vi "NT Writer.vi"() -> ()   [LabVIEW 2015]
uses:
  NT Variable TypeDef.ctl
  <vilib>/Rock Robotics/Network Tables/NT Write Number.vi
  <vilib>/Rock Robotics/Network Tables/NT Write Boolean.vi
  <vilib>/Rock Robotics/Network Tables/NT Write String.vi
  <vilib>/Rock Robotics/Network Tables/NT Write Boolean Array.vi
  <vilib>/Rock Robotics/Network Tables/NT Write Numeric Array.vi
  <vilib>/Rock Robotics/Network Tables/NT Write String Array.vi
panel:
  in  "Write":bool
  in  "PID":cluster{"Kp":dbl, "Ki":dbl, "Kd":dbl}
  in  "String Array":string[](array[string])
  in  "String":string
  in  "Numeric Array":dbl[](array[numeric])
  in  "Numeric":dbl
  in  "Boolean Array":bool[](array[boolean])
  in  "stop":bool
  in  "Boolean":bool
  in  "NT Variable":u16(ring) items=["/Robot Parameters/Arm Parameters/Position Sensor Calibration/Voltage @ Max Angle (v)", "/Robot Parameters/Arm Parameters/Position Sensor Calibration/Voltage @ Min Angle (v)", "/Robot Parameters/Arm Parameters/Position Sensor Calibration/Max Angle (°)", "/Robot Parameters/Arm Parameters/Position Sensor Calibration/Min Angle (°)", "/Robot Parameters/Arm Parameters/Arm angle tolerance to lock (+|-°)", "/Robot Parameters/Drive Parameters/Default Orientation (F-Normal; T-Reversed)", "/Robot Parameters/Intake Parameters/Suck-in Speed (-1 to 1)", "/Robot Parameters/Intake Parameters/Spit-out Speed (-1 to 1)", "/Robot Parameters/Arm Parameters/Auto Arm Up Speed (in per s)", "/Robot Parameters/Arm Parameters/Position Sensor Calibration/Min Angle (°)", "/Robot Parameters/Arm Parameters/Position Sensor Calibration/Max Angle (°)", "/Robot Parameters/Arm Parameters/Driver Cross Defense Angle  (90° - 180°)", "/Robot Parameters/Drive Parameters/Reduced Speed Gain (0-1)", "/Robot Parameters/Arm Parameters/Arm Motor PID Gains", "/Robot Parameters/Shooter Parameters/Shoot Solenoid Time (ms)", "/Robot Parameters/Shooter Parameters/Open Claw Time (ms)", "/Robot Parameters/Shooter Parameters/Pressure threshold for shooting (PSI)", "/Robot Parameters/Drive Parameters/IMU PID Gains", "/Robot Parameters/Drive Parameters/Encoder PID Gains", "/Robot Parameters/Drive Parameters/GRIP PID Gains", "/Robot Parameters/Shooter Parameters/Arm angle threshold for shooting (90°-180°)", "/Robot Parameters/Drive Parameters/Slew Rate (Units per Second)", "/Robot Parameters/Drive Parameters/Joystick Configuration (0 - Split Axis Arcade; 1 - Arcade; 2 - Tank)", "/Robot Parameters/Arm Parameters/Presets/Shoot Batter (°, Lock)", "/Robot Parameters/Arm Parameters/Presets/Shoot Close (°, Lock)", "/Robot Parameters/Arm Parameters/Presets/Cross Defense (°, Lock)", "/Robot Parameters/Arm Parameters/Presets/Human Player Load (°, Lock)", "/Robot Parameters/Arm Parameters/Presets/Low Bar, Low Goal (°, Lock)"]
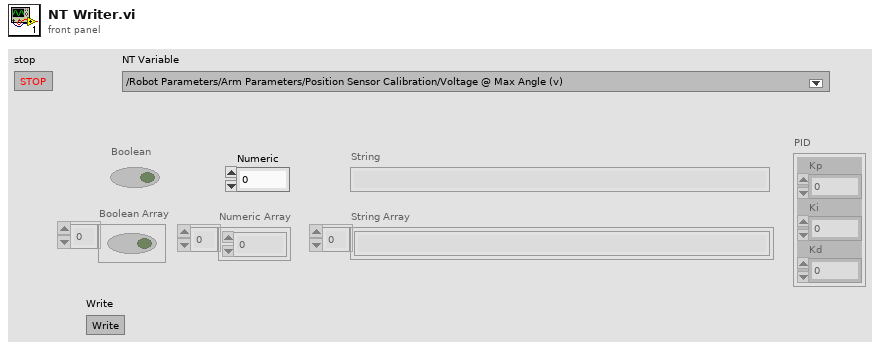
[diagram p1: front panel]
types:
  T1 = typedef "NT Variable TypeDef.ctl" = cluster{"NT Variable Name":string, "NT Type":enum16{"Boolean", "Numeric", "String", "Boolean Array", "Numeric Array", "String Array", "PID"}}
  T2 = enum8{"Enabled", "Disabled", "Disabled and Grayed Out"}
  T3 = enum16{"Boolean", "Numeric", "String", "Boolean Array", "Numeric Array", "String Array", "PID"}
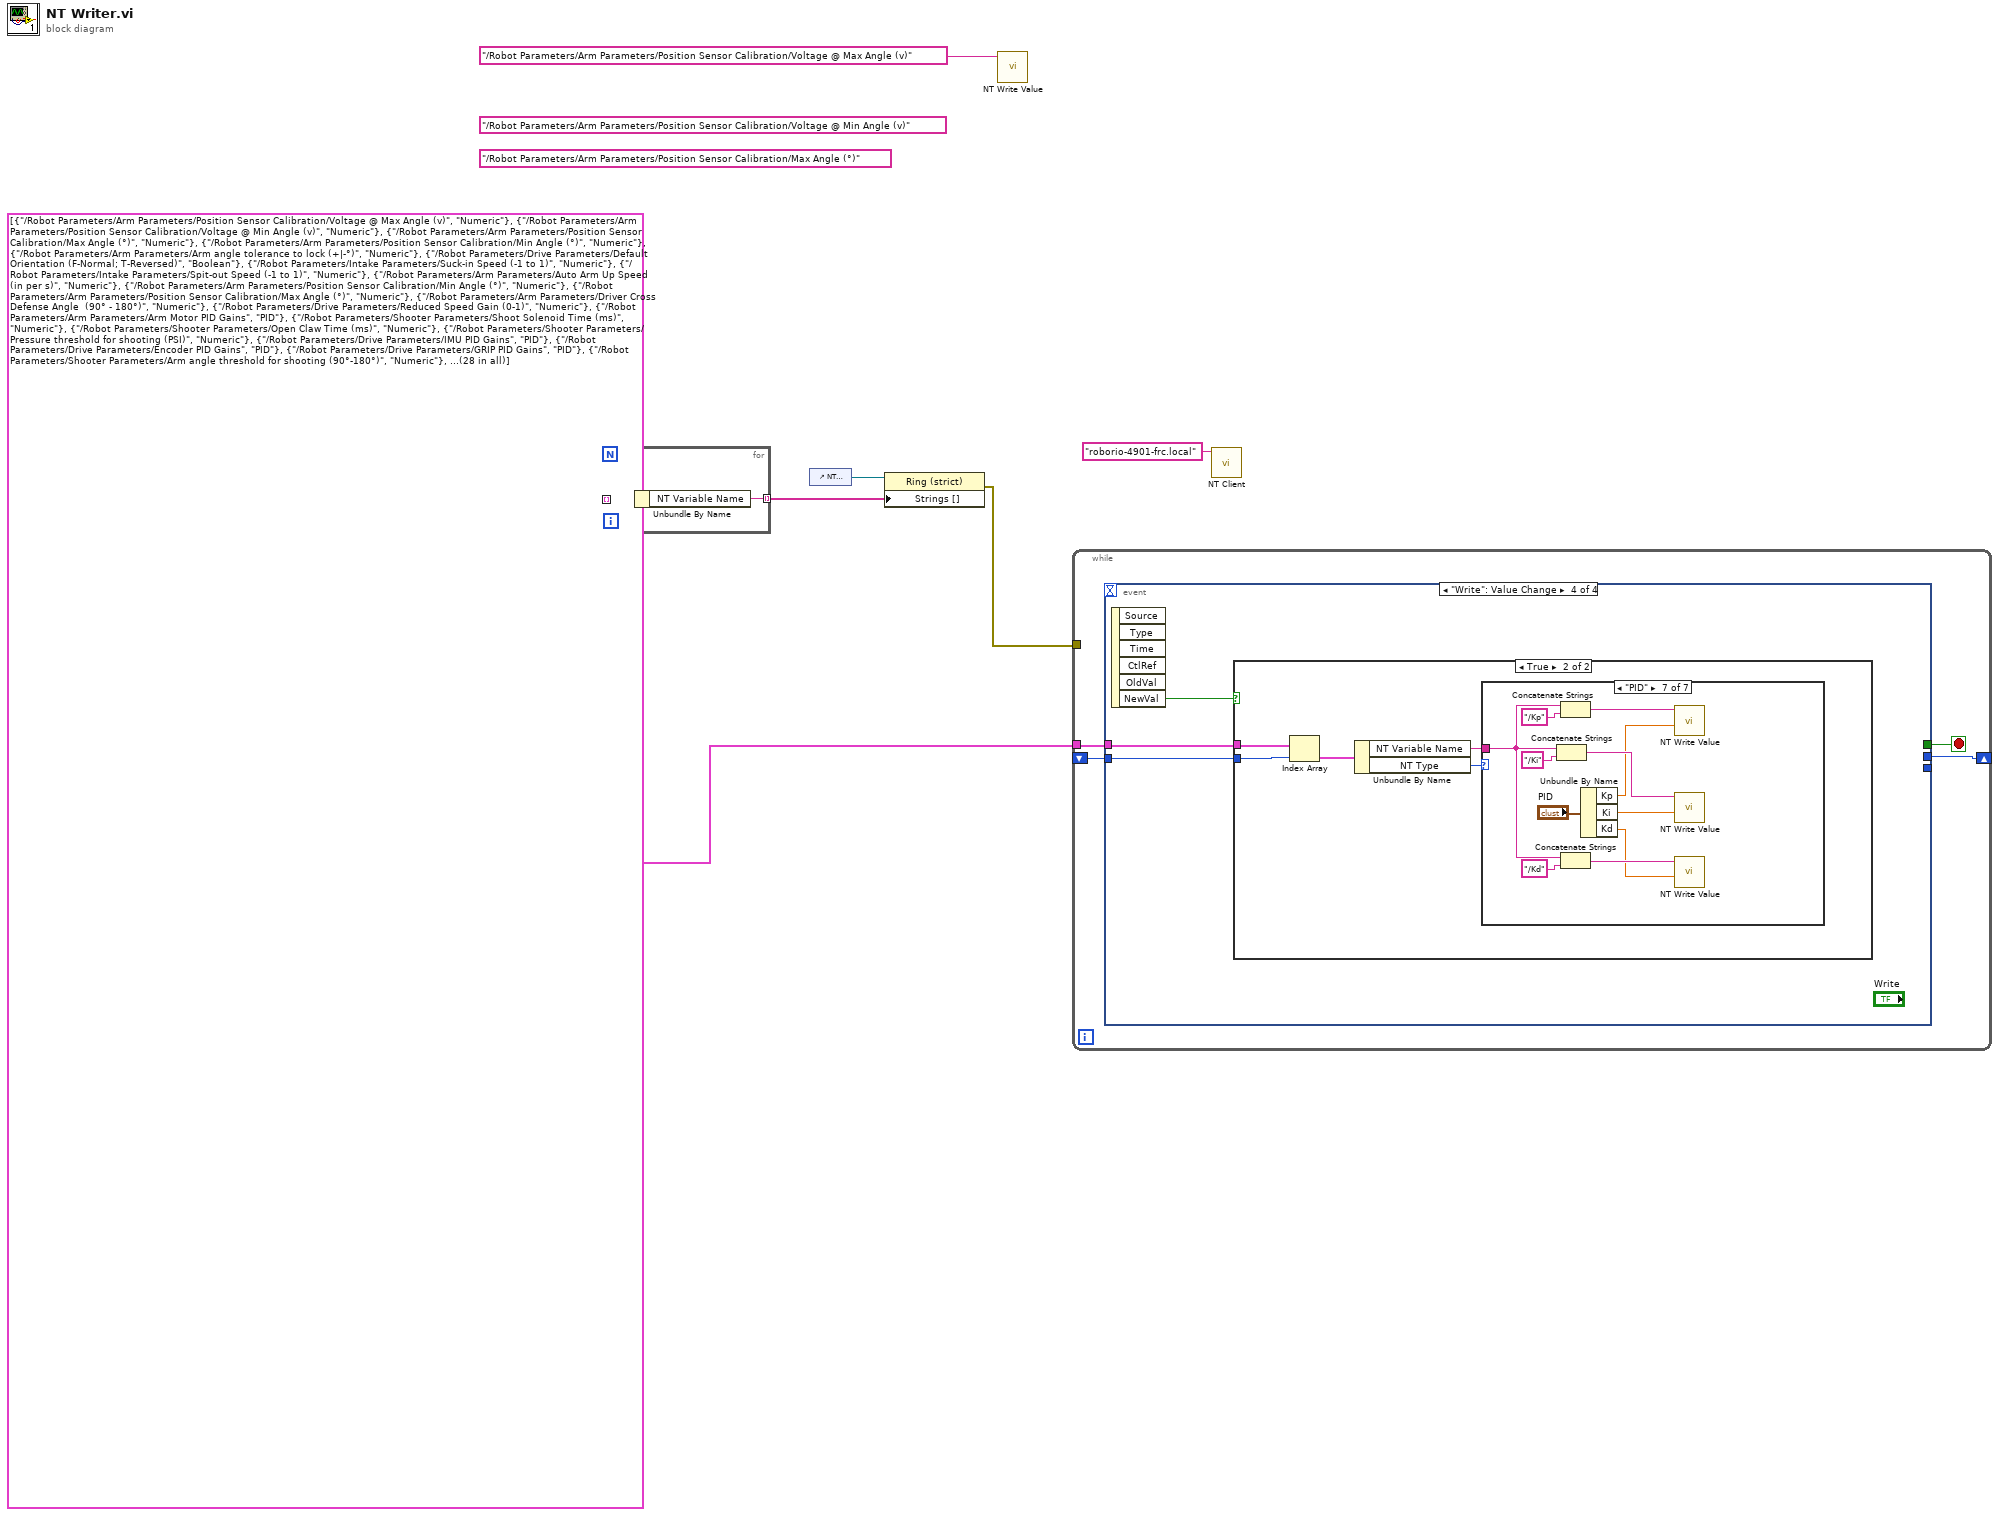
[diagram p0: block diagram]
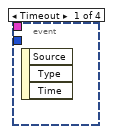
[diagram p2: hidden frame]
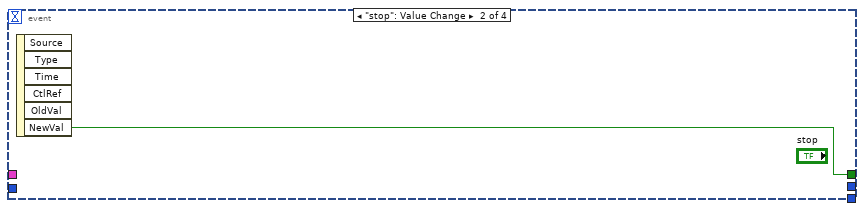
[diagram p3: hidden frame]
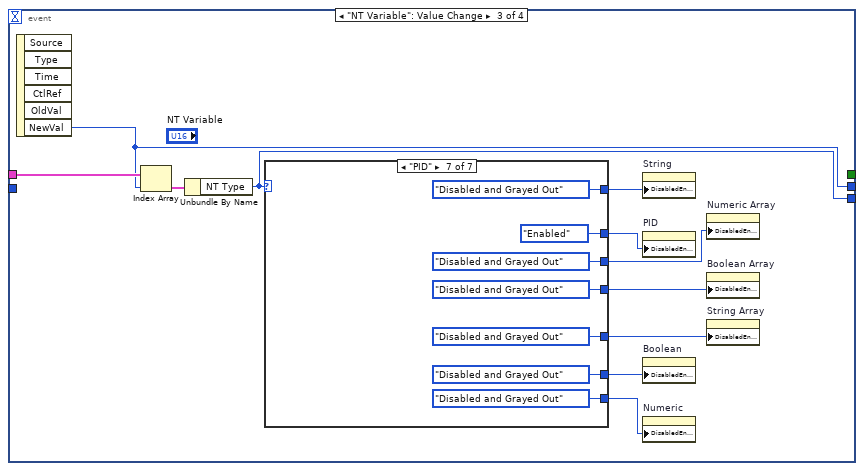
[diagram p4: hidden frame]
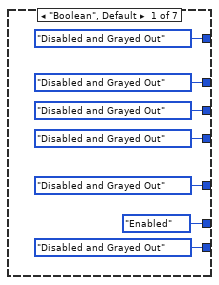
[diagram p5: hidden frame]
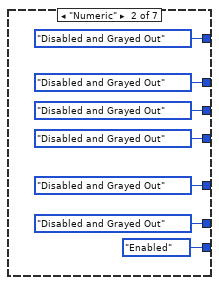
[diagram p6: hidden frame]
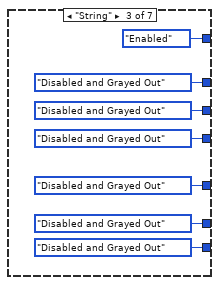
[diagram p7: hidden frame]
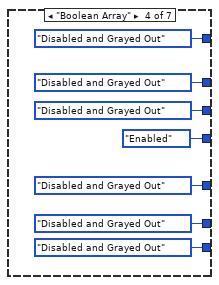
[diagram p8: hidden frame]
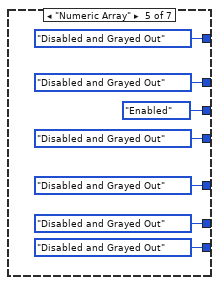
[diagram p9: hidden frame]
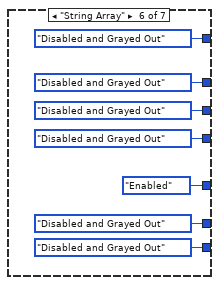
[diagram p10: hidden frame]
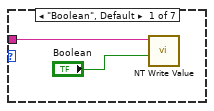
[diagram p12: hidden frame]
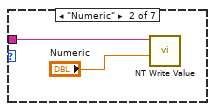
[diagram p13: hidden frame]
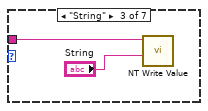
[diagram p14: hidden frame]
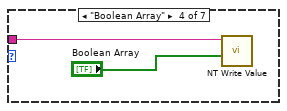
[diagram p15: hidden frame]
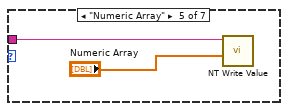
[diagram p16: hidden frame]
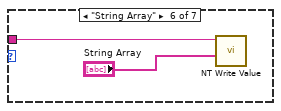
[diagram p17: hidden frame]
diagram:
  w3 = T1[] [{"NT Variable Name"="/Robot Parameters/Arm Parameters/Position Sensor Calibration/Voltage @ Max Angle (v)", "NT Type"=enum."Numeric"}, {"NT Variable Name"="/Robot Parameters/Arm Parameters/Position Sensor Calibration/Voltage @ Min Angle (v)", "NT Type"=enum."Numeric"}, {"NT Variable Name"="/Robot Parameters/Arm Parameters/Position Sensor Calibration/Max Angle (°)", "NT Type"=enum."Numeric"}, {"NT Variable Name"="/Robot Parameters/Arm Parameters/Position Sensor Calibration/Min Angle (°)", "NT Type"=enum."Numeric"}, {"NT Variable Name"="/Robot Parameters/Arm Parameters/Arm angle tolerance to lock (+|-°)", "NT Type"=enum."Numeric"}, {"NT Variable Name"="/Robot Parameters/Drive Parameters/Default Orientation (F-Normal; T-Reversed)", "NT Type"=enum."Boolean"}, {"NT Variable Name"="/Robot Parameters/Intake Parameters/Suck-in Speed (-1 to 1)", "NT Type"=enum."Numeric"}, {"NT Variable Name"="/Robot Parameters/Intake Parameters/Spit-out Speed (-1 to 1)", "NT Type"=enum."Numeric"}, {"NT Variable Name"="/Robot Parameters/Arm Parameters/Auto Arm Up Speed (in per s)", "NT Type"=enum."Numeric"}, {"NT Variable Name"="/Robot Parameters/Arm Parameters/Position Sensor Calibration/Min Angle (°)", "NT Type"=enum."Numeric"}, {"NT Variable Name"="/Robot Parameters/Arm Parameters/Position Sensor Calibration/Max Angle (°)", "NT Type"=enum."Numeric"}, {"NT Variable Name"="/Robot Parameters/Arm Parameters/Driver Cross Defense Angle  (90° - 180°)", "NT Type"=enum."Numeric"}, {"NT Variable Name"="/Robot Parameters/Drive Parameters/Reduced Speed Gain (0-1)", "NT Type"=enum."Numeric"}, {"NT Variable Name"="/Robot Parameters/Arm Parameters/Arm Motor PID Gains", "NT Type"=enum."PID"}, {"NT Variable Name"="/Robot Parameters/Shooter Parameters/Shoot Solenoid Time (ms)", "NT Type"=enum."Numeric"}, {"NT Variable Name"="/Robot Parameters/Shooter Parameters/Open Claw Time (ms)", "NT Type"=enum."Numeric"}, {"NT Variable Name"="/Robot Parameters/Shooter Parameters/Pressure threshold for shooting (PSI)", "NT Type"=enum."Numeric"}, {"NT Variable Name"="/Robot Parameters/Drive Parameters/IMU PID Gains", "NT Type"=enum."PID"}, {"NT Variable Name"="/Robot Parameters/Drive Parameters/Encoder PID Gains", "NT Type"=enum."PID"}, {"NT Variable Name"="/Robot Parameters/Drive Parameters/GRIP PID Gains", "NT Type"=enum."PID"}, {"NT Variable Name"="/Robot Parameters/Shooter Parameters/Arm angle threshold for shooting (90°-180°)", "NT Type"=enum."Numeric"}, {"NT Variable Name"="/Robot Parameters/Drive Parameters/Slew Rate (Units per Second)", "NT Type"=enum."Numeric"}, {"NT Variable Name"="/Robot Parameters/Drive Parameters/Joystick Configuration (0 - Split Axis Arcade; 1 - Arcade; 2 - Tank)", "NT Type"=enum."Numeric"}, {"NT Variable Name"="/Robot Parameters/Arm Parameters/Presets/Shoot Batter (°, Lock)", "NT Type"=enum."String"}, {"NT Variable Name"="/Robot Parameters/Arm Parameters/Presets/Shoot Close (°, Lock)", "NT Type"=enum."String"}, {"NT Variable Name"="/Robot Parameters/Arm Parameters/Presets/Cross Defense (°, Lock)", "NT Type"=enum."String"}, {"NT Variable Name"="/Robot Parameters/Arm Parameters/Presets/Human Player Load (°, Lock)", "NT Type"=enum."String"}, {"NT Variable Name"="/Robot Parameters/Arm Parameters/Presets/Low Bar, Low Goal (°, Lock)", "NT Type"=enum."String"}]
  (unwired) "/Robot Parameters/Arm Parameters/Position Sensor Calibration/Max Angle (°)" ("Name")
  (unwired) "/Robot Parameters/Arm Parameters/Position Sensor Calibration/Voltage @ Min Angle (v)" ("Name")
  n1 = for {
    tunnel: w3 -> [w8] mode=indexing
    tunnel: [w7] -> w4 mode=indexing
    n2 = Unbundle By Name(w8) -> ("NT Variable Name"=w7:string)
  }
  n3 = control-ref of="NT Variable"() -> (w5:refnum<vi>)
  n4 = property class="Ring (strict)"(reference=w5, "Strings []"=w4) -> (error out=w2:errorcluster)  [unwired: 1 in, 1 out]
  n5 = call-poly <vilib>:"NT Write Value.vi"("Name"="/Robot Parameters/Arm Parameters/Position Sensor Calibration/Voltage @ Max Angle (v)") -> ()  [unwired: 10 in, 1 out]
  n6 = while {
    tunnel: w3 -> [w12]
    shift-right: [w10] -> _
    shift-left: _ -> [w9]
    tunnel: w2 -> [_]
    stop <- w11 stop-if-true
    n7 = event shown="[3] \"Write\": Value Change" {
      selector: _ -> [_ _ _ _]
      dyn-events: _ -> [_ _ _ _]
      timeout: _ -> [_ _ _ _]
      tunnel: w12 -> [_ _ w23 w75]
      tunnel: [_ w13 _ _] -> w11
      tunnel: [_ _ w15 _] -> _
      tunnel: [_ _ w14 _] -> w10
      tunnel: w9 -> [_ _ _ w74]
      event Timeout {
        n8 = event-data() -> ()  [unwired: 1 in, 3 out]
      }
      event "stop": Value Change {
        n9 = event-data() -> ("NewVal"=w13:bool)  [unwired: 1 in, 5 out]
      }
      event "NT Variable": Value Change {
        n10 = event-data() -> ("NewVal"=w14:u16)  [unwired: 1 in, 5 out]
        n11 = Index Array(array=w23, index=w14) -> (element=w24:T1)
        n12 = Unbundle By Name(w24) -> ("NT Type"=w15:T3)
        n13 = case shown="\"PID\"" w15 {
          tunnel: [T2."Enabled" ("Disabled") T2."Disabled and Grayed Out" ("Disabled") T2."Disabled and Grayed Out" ("Disabled") T2."Disabled and Grayed Out" ("Disabled") T2."Disabled and Grayed Out" ("Disabled") T2."Disabled and Grayed Out" ("Disabled") T2."Disabled and Grayed Out" ("Disabled")] -> w22
          tunnel: [T2."Disabled and Grayed Out" ("Disabled") T2."Disabled and Grayed Out" ("Disabled") T2."Disabled and Grayed Out" ("Disabled") T2."Disabled and Grayed Out" ("Disabled") T2."Disabled and Grayed Out" ("Disabled") T2."Disabled and Grayed Out" ("Disabled") T2."Enabled" ("Disabled")] -> w21
          tunnel: [T2."Disabled and Grayed Out" ("Disabled") T2."Disabled and Grayed Out" ("Disabled") T2."Disabled and Grayed Out" ("Disabled") T2."Disabled and Grayed Out" ("Disabled") T2."Disabled and Grayed Out" ("Disabled") T2."Enabled" ("Disabled") T2."Disabled and Grayed Out" ("Disabled")] -> w20
          tunnel: [T2."Disabled and Grayed Out" ("Disabled") T2."Disabled and Grayed Out" ("Disabled") T2."Disabled and Grayed Out" ("Disabled") T2."Disabled and Grayed Out" ("Disabled") T2."Enabled" ("Disabled") T2."Disabled and Grayed Out" ("Disabled") T2."Disabled and Grayed Out" ("Disabled")] -> w19
          tunnel: [T2."Disabled and Grayed Out" ("Disabled") T2."Disabled and Grayed Out" ("Disabled") T2."Disabled and Grayed Out" ("Disabled") T2."Enabled" ("Disabled") T2."Disabled and Grayed Out" ("Disabled") T2."Disabled and Grayed Out" ("Disabled") T2."Disabled and Grayed Out" ("Disabled")] -> w18
          tunnel: [T2."Disabled and Grayed Out" ("Disabled") T2."Disabled and Grayed Out" ("Disabled") T2."Enabled" ("Disabled") T2."Disabled and Grayed Out" ("Disabled") T2."Disabled and Grayed Out" ("Disabled") T2."Disabled and Grayed Out" ("Disabled") T2."Disabled and Grayed Out" ("Disabled")] -> w17
          tunnel: [T2."Disabled and Grayed Out" ("Disabled") T2."Enabled" ("Disabled") T2."Disabled and Grayed Out" ("Disabled") T2."Disabled and Grayed Out" ("Disabled") T2."Disabled and Grayed Out" ("Disabled") T2."Disabled and Grayed Out" ("Disabled") T2."Disabled and Grayed Out" ("Disabled")] -> w16
          frame "Boolean", Default {
          }
          frame "Numeric" {
          }
          frame "String" {
          }
          frame "Boolean Array" {
          }
          frame "Numeric Array" {
          }
          frame "String Array" {
          }
          frame "PID" {
          }
        }
        n14 = property on="String" class="Str"("DisabledEnum"=w17) -> ()  [unwired: 2 in, 2 out]
        n15 = property on="PID" class="Clust (strict)"("DisabledEnum"=w21) -> ()  [unwired: 2 in, 2 out]
        n16 = property on="Boolean" class="Bool (strict)"("DisabledEnum"=w22) -> ()  [unwired: 2 in, 2 out]
        n17 = property on="Numeric" class="DigNum (strict)"("DisabledEnum"=w16) -> ()  [unwired: 2 in, 2 out]
        n18 = property on="Numeric Array" class="Arr (strict)"("DisabledEnum"=w19) -> ()  [unwired: 2 in, 2 out]
        n19 = property on="Boolean Array" class="Arr (strict)"("DisabledEnum"=w18) -> ()  [unwired: 2 in, 2 out]
        n20 = property on="String Array" class="Arr (strict)"("DisabledEnum"=w20) -> ()  [unwired: 2 in, 2 out]
      }
      event "Write": Value Change {
        n21 = event-data() -> ("NewVal"=w76:bool)  [unwired: 1 in, 5 out]
        n22 = case shown="True" w76 {
          tunnel: w75 -> [_ w81]
          tunnel: w74 -> [_ w80]
          frame False {
          }
          frame True {
            n23 = Index Array(array=w81, index=w80) -> (element=w79:T1)
            n24 = Unbundle By Name(w79) -> ("NT Variable Name"=w77:string, "NT Type"=w78:T3)
            n25 = case shown="\"PID\"" w78 {
              tunnel: w77 -> [w82 w85 w87 w89 w91 w93 w101]
              frame "Boolean", Default {
                n26 = call-poly <vilib>:"NT Write Value.vi"("Boolean"="Boolean", "Name"=w82) -> ()  [unwired: 9 in, 1 out]
              }
              frame "Numeric" {
                n27 = call-poly <vilib>:"NT Write Value.vi"("Numeric"="Numeric", "Name"=w85) -> ()  [unwired: 9 in, 1 out]
              }
              frame "String" {
                n28 = call-poly <vilib>:"NT Write Value.vi"("String"="String", "Name"=w87) -> ()  [unwired: 9 in, 1 out]
              }
              frame "Boolean Array" {
                n29 = call-poly <vilib>:"NT Write Value.vi"("Boolean Array"="Boolean Array", "Name"=w89) -> ()  [unwired: 9 in, 1 out]
              }
              frame "Numeric Array" {
                n30 = call-poly <vilib>:"NT Write Value.vi"("Numeric Array"="Numeric Array", "Name"=w91) -> ()  [unwired: 9 in, 1 out]
              }
              frame "String Array" {
                n31 = call-poly <vilib>:"NT Write Value.vi"("String Array"="String Array", "Name"=w93) -> ()  [unwired: 9 in, 1 out]
              }
              frame "PID" {
                n32 = Concatenate Strings(w101, "/Ki" ("string")) -> (w98:string)
                n33 = Concatenate Strings(w101, "/Kp" ("string")) -> (w97:string)
                n34 = Concatenate Strings(w101, "/Kd" ("string")) -> (w99:string)
                n35 = Unbundle By Name("PID") -> ("Kp"=w96:dbl, "Ki"=w95:dbl, "Kd"=w94:dbl)
                n36 = call-poly <vilib>:"NT Write Value.vi"("Numeric"=w96, "Name"=w97) -> ()  [unwired: 9 in, 1 out]
                n37 = call-poly <vilib>:"NT Write Value.vi"("Numeric"=w95, "Name"=w98) -> ()  [unwired: 9 in, 1 out]
                n38 = call-poly <vilib>:"NT Write Value.vi"("Numeric"=w94, "Name"=w99) -> ()  [unwired: 9 in, 1 out]
              }
            }
          }
        }
      }
    }
  }
  n39 = call <vilib>:"NT Client.vi"("Server IP Address"="roborio-4901-frc.local") -> ()  [unwired: 11 in]
